vi "Update Pre-Trigger Samples in Record.vi"(8 "Increment?":bool, 9 "Pre-Trigger Samples Acquired":u16, 11 "Pre-Trigger Samples to Acquire":u16) -> (0 "Pre-Trigger Samples Done ?":bool, 1 "Updated Pre-Trigger Samples Done":u16, 2 "Is Pre-Trig =0?":bool, 3 "Pre-Trigger Samples to Acquire":u16)   [LabVIEW 2012]
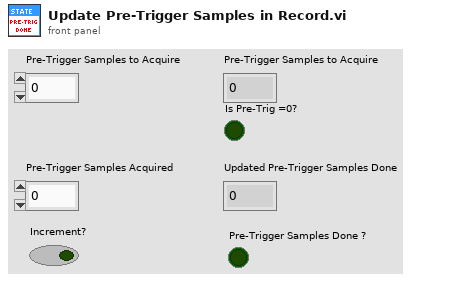
[diagram p1: front panel]
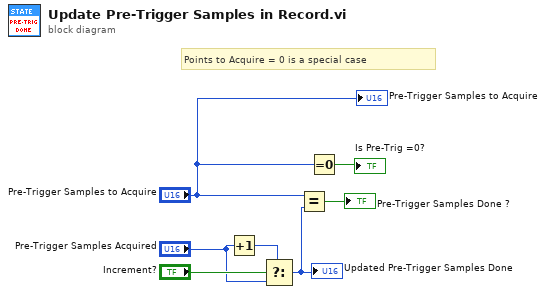
[diagram p0: block diagram]
diagram:
  # "Points to Acquire = 0 is a special case"
  n1 = Increment(x="Pre-Trigger Samples Acquired") -> (x+1=w7:u16)
  n2 = Select(t=w7, s="Increment?", f="Pre-Trigger Samples Acquired") -> (s? t:f=w4:u16)
  "Updated Pre-Trigger Samples Done" <- w4
  n3 = Equal?(x="Pre-Trigger Samples to Acquire", y=w4) -> (x = y?=→"Pre-Trigger Samples Done ?":bool)
  n4 = Equal To 0?(x="Pre-Trigger Samples to Acquire") -> (x = 0?=→"Is Pre-Trig =0?":bool)
  "Pre-Trigger Samples to Acquire" <- "Pre-Trigger Samples to Acquire"
